vi "ReadCSV.vi"() -> ()   [LabVIEW 2017]
uses:
  <vilib>/Utility/file.llb/Read Delimited Spreadsheet (I64).vi
panel:
  out "all rows":i64[][](array[numeric])
  out "z":i64
  out "y":i64
  out "x":i64
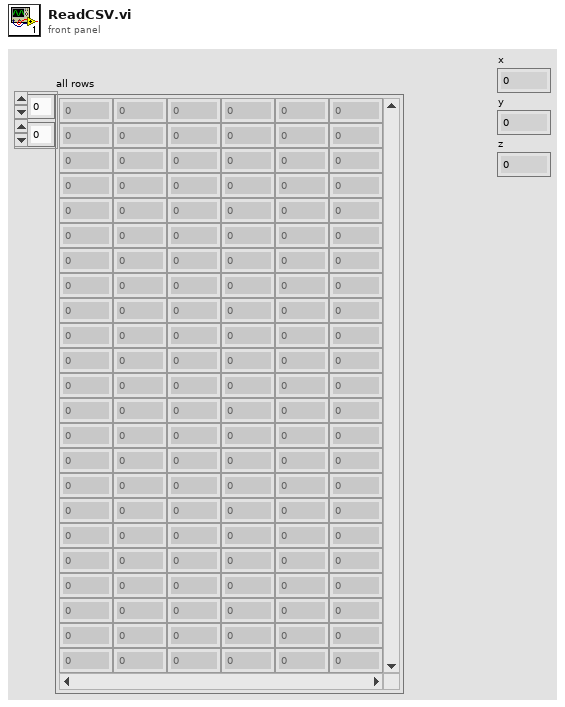
[diagram p1: front panel]
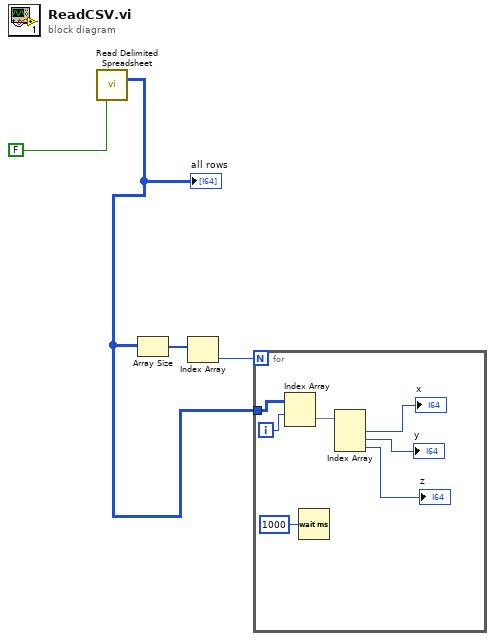
[diagram p0: block diagram]
diagram:
  n1 = call-poly <vilib>:"Read Delimited Spreadsheet.vi"("transpose? (F)"=FALSE) -> ("all rows"=w3:i64[][])  [unwired: 9 in, 5 out]
  "all rows" <- w3
  n2 = Array Size(array=w3) -> (size(s)=w2:i32[])
  n3 = Index Array(array=w2) -> (element=w1:i32)  [unwired: 1 in]
  n4 = for {
    N: w1 -> [_]
    tunnel: w3 -> [w7]
    i -> [w5]
    n5 = Index Array(array=w7, index (row)=w5) -> (element=w6:i64[])  [unwired: 1 in]
    n6 = Wait (ms)(milliseconds to wait=u32 1000) -> ()  [unwired: 1 out]
    n7 = Index Array(array=w6) -> (element #1=→"x":i64, element #2=→"y":i64, element #3=→"z":i64)  [unwired: 3 in]
  }
